vi "GlobalVariables.vi"() -> ()   [LabVIEW 2016]
panel:
  out "stopReading":bool
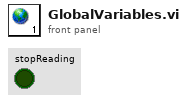
[diagram p1: front panel]
diagram:
